vi "RT Main.vi"() -> ()   [LabVIEW 2017]
doc: "The myRIO Custom FPGA Project template acquires button data from the onboard button and displays the button value on a Boolean indicator. The SYS.RDY indicator shows the FPGA status."
uses:
  <vilib>/Platform/TimedLoop/XDataNode/timing_clust.ctl
  <vilib>/Platform/TimedLoop/XDataNode/nitl_modes.ctl
  <vilib>/Platform/TimedLoop/XDataNode/wakeup.ctl
  <vilib>/FPGAPlugInAG/myRIO-1900/niLvFpga_Open_myRIO-1900.vi
  <vilib>/rvi/interface/common/dynamic/niFpgaDynamicAddResources.vi
  <vilib>/myRIO/Common/Instrument Driver Framework/Utilities/vis/FPGA Ref Manager.vi
  <vilib>/Utility/error.llb/Error Cluster From Error Code.vi
  <vilib>/myRIO/Common/Instrument Driver Framework/Utilities/vis/Ref Counter.vi
  <vilib>/rvi/errors/niLvFpgaAdjustHostInterfaceError.vi
  <vilib>/FPGAPlugInAG/Dynamic/niLvFpga_Close_Dynamic.vi
  <vilib>/rvi/interface/nirviOpenFPGA/nirviOpenFPGA.xnode
  FPGA Bitfiles/FPGADEMO_FPGATarget_FPGAENCODER_OUiAhW3lqQo.lvbitx
  FPGA ENCODER.vi
  <vilib>/platform/TimedLoop/XDataNode/XDataNode.xnode
  <vilib>/rvi/interface/nirviReadWriteControl/nirviReadWriteControl.xnode
  <vilib>/rvi/interface/nirviCloseFPGA/nirviCloseFPGA.xnode
  <vilib>/myRIO/Instrument Drivers/Utilities/Utilities.lvlib
  NiFpgaLv.dll
  <vilib>/rvi/interface/Simulation/niFpgaSimulationCallBeginRW.vi
  <vilib>/Platform/TimedLoop/XDataNode/XDNodeRunTimeDep.lvlib
panel:
  out "Waveform Chart":dbl[](graph)
  out "error out":errorcluster
  in  "Filter Counts":u16
  in  "Clear Overflow?":bool
  in  "Clear Error?":bool
  in  "Reset":bool
  in  "Stop":bool
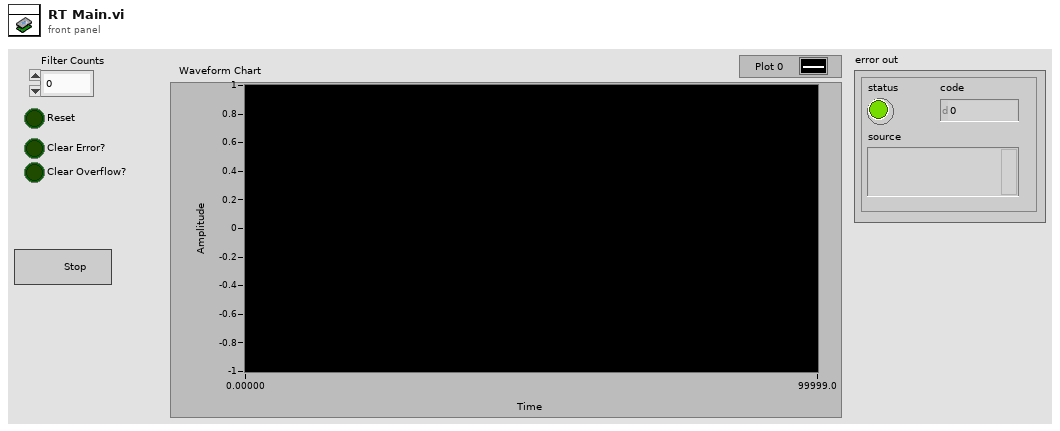
[diagram p1: front panel]
types:
  T1 = typedef "XDNodeRunTimeDep.lvlib/timing_clust.ctl" = cluster{"Expected End [f-1]":u64, "Actual End [f-1]":u64, "Finished Late? [f-1]":bool, "Expected End [i-1]":u64, "Actual End [i-1]":u64, "Finished Late? [i-1]":bool, "Expected Start [i]":u64, "Actual Start [i]":u64, "Expected Start [f]":u64, "Actual Start [f]":u64, "Source Name":string, "Structure Name":string, "Period":i64, "Deadline":i64, "Offset":i64, "Start":i64, "Priority":i32, "Timeout":i32, "Mode":T2, "Wakeup Reason":T3, "Error":errorcluster, "Source Type":string, "Secondary Source Type":string, "Global End Time":u64, "Global Start Time":u64, "Frame Duration":u64, "Iteration Duration":u64, "Assigned CPU":i32, "I/O Scan Engine Mode":u32}
  T2 = typedef "XDNodeRunTimeDep.lvlib/nitl_modes.ctl" = enum32{"No Change", "Process missed periods, maintain original phase", "Discard missed periods, maintain original phase", "Process missed periods, ignore original phase", "Discard missed periods, ignore original phase"}
  T3 = typedef "XDNodeRunTimeDep.lvlib/wakeup.ctl" = enum32{"Normal", "Aborted", "Asynchronous wakeup", "Timing source error", "Timed loop error", "Timeout"}
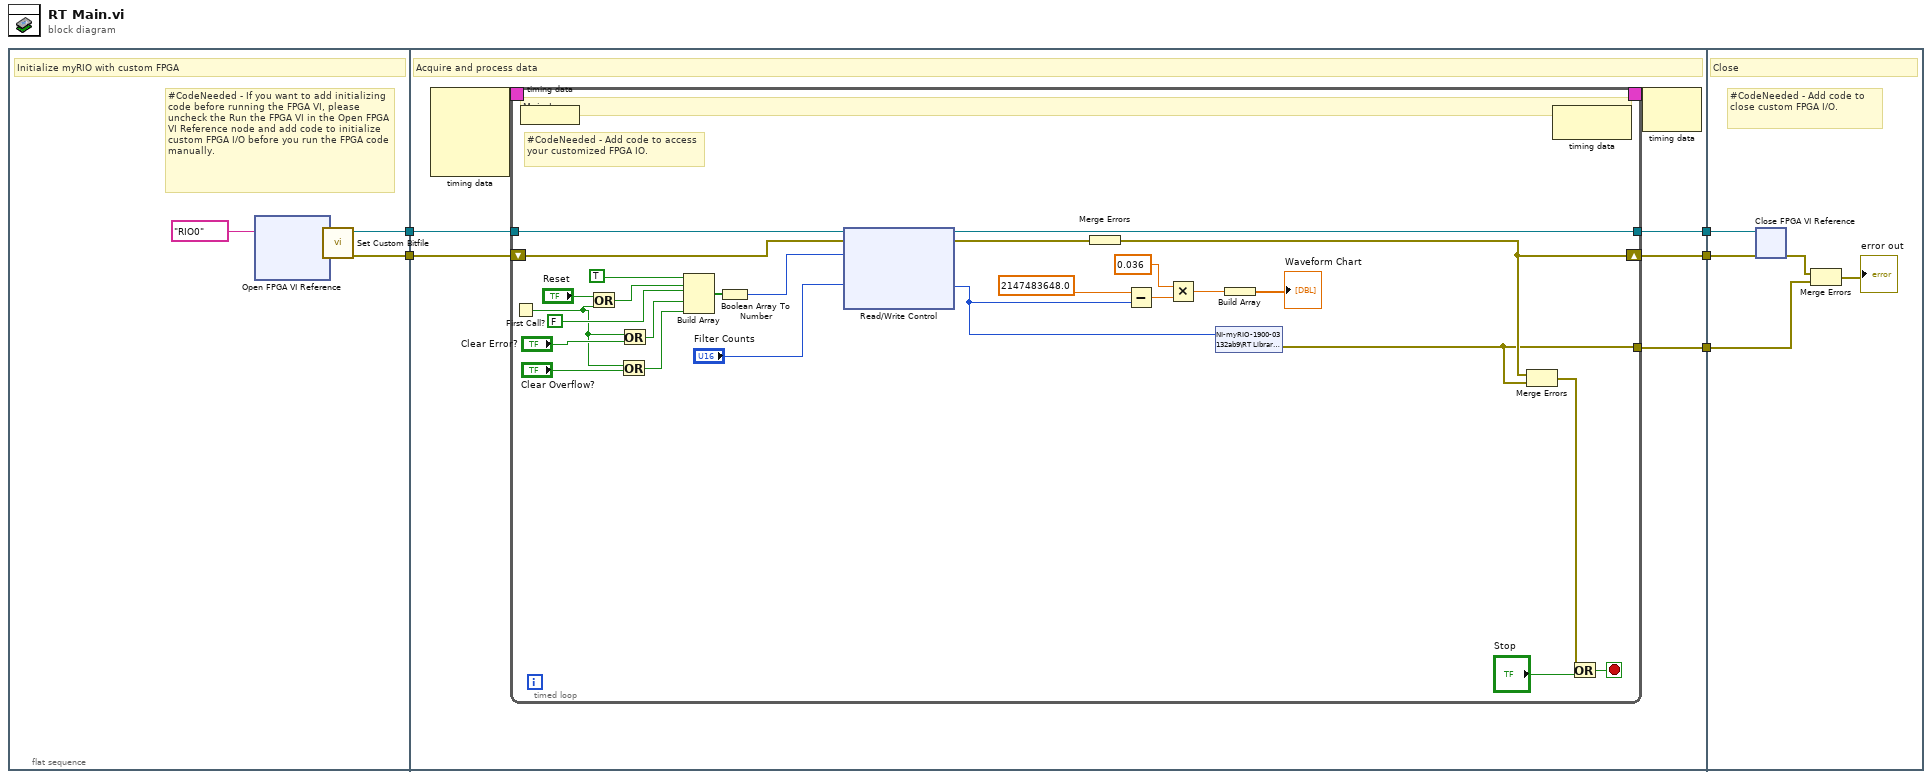
[diagram p0: block diagram]
diagram:
  n1 = flat-sequence {
    tunnel: [w6] -> w5
    tunnel: [w7] -> w4
    tunnel: w5 -> [w17]
    tunnel: w4 -> [w16]
    tunnel: [w15] -> w3
    tunnel: [w14] -> w2
    tunnel: [w11] -> w1
    tunnel: w3 -> [w53]
    tunnel: w2 -> [w52]
    tunnel: w1 -> [w49]
    frame #0 {
      # "#CodeNeeded - If you want to add initializing code before running the FPGA VI, please uncheck the Run the FPGA VI in the Open FPGA VI Reference node and add code to initialize custom FPGA I/O before you run the FPGA code manually."
      # "Initialize myRIO with custom FPGA"
      n2 = xnode "Open FPGA VI Reference"("resource name"=tag "RIO0") -> ("FPGA VI Reference Out"=w8:refnum<k20>, "error out"=w9:errorcluster)  [unwired: 1 in]
      n3 = call <vilib>:"Set Custom Bitfile.vi"("error in (no error)"=w9, "Custom FPGA Reference In"=w8) -> ("error out"=w6:errorcluster, "Custom FPGA Reference Out"=w7:refnum<k20>)  [unwired: 8 in]
    }
    frame #1 {
      # "Acquire and process data"
      n4 = node-c288() -> (w13:T1)  [unwired: 4 in]
      n5 = timed-loop {
        tunnel: w16 -> [w42]
        tunnel: [w41] -> w15
        shift-right: [w26] -> w14
        shift-left: w17 -> [w39]
        timing: w13 -> [_]
        timing-out: [_] -> w12
        tunnel: [w24] -> w11
        stop <- w43 stop-if-true
        # "#CodeNeeded - Add code to access your customized FPGA IO."
        # "Main Loop"
        n6 = First Call?() -> (First Call?: T/F=w28:bool)
        n7 = node-c288() -> ()  [unwired: 1 in]
        n8 = Or(x="Reset", y=w28) -> (x .or. y?=w37:bool)
        n9 = Or(x=w28, y="Clear Overflow?") -> (x .or. y?=w30:bool)
        n10 = Or(x=w28, y="Clear Error?") -> (x .or. y?=w32:bool)
        n11 = Build Array(TRUE, w37, FALSE, w32, w30) -> (w36:bool[])
        n12 = Boolean Array To Number(Boolean array=w36) -> (number=w35:u32)
        n13 = xnode "Read/Write Control"("FPGA VI Reference In"=w42, "error in"=w39, "CNFG"=w35, "Debounce Ticks"="Filter Counts") -> ("FPGA VI Reference Out"=w41:refnum<k20>, "error out"=w40:errorcluster, "CNTR"=w20:u32)  [unwired: 1 out]
        n14 = Merge Errors(w40) -> (w26:errorcluster)
        n15 = Subtract(x=2147483648.0, y=w20) -> (x-y=w23:dbl)
        n16 = Multiply(x=0.036, y=w23) -> (x*y=w19:dbl)
        n17 = shared-variable "NI-myRIO-1900-03132ab9\\RT Library.lvlib\\SV2"(w20) -> (error out=w24:errorcluster)  [unwired: 1 in]
        n18 = Build Array(w19) -> (→"Waveform Chart":dbl[])
        n19 = Merge Errors(w26, w24) -> (w25:errorcluster)
        n20 = node-c288() -> ()  [unwired: 1 in, 1 out]
        n21 = Or(x=w25, y="Stop") -> (x .or. y?=w43:bool)
      }
      n22 = node-c288(w12) -> ()  [unwired: 1 out]
    }
    frame #2 {
      # "#CodeNeeded - Add code to close custom FPGA I/O."
      # "Close"
      n23 = xnode "Close FPGA VI Reference"("FPGA VI Reference In"=w53, "error in"=w52) -> ("error out"=w51:errorcluster)
      n24 = Merge Errors(w51, w49) -> (→"error out":errorcluster)
    }
  }
